vi "Ruler.vi"() -> ()   [LabVIEW 2023]
uses:
  <vilib>/measure/matone.llb/Extract Single Tone Information N Chan.vi
  <vilib>/express/express analysis/Spectral/Block/exnSpectralBlock spectral measurements RMS poly.vi
  <vilib>/express/express analysis/Spectral/Block/exnSpectralBlock spectral measurements RMS DDT.vi
  <vilib>/express/express analysis/Spectral/XNode/ExpressSpectralMeasurementsBlockNode.xnode
  <vilib>/measure/NI_MAPro.lvlib
panel:
  out "Waveform Chart of Acquired Sound":dynamicdata(graph) caption="Data"
  out "Fundamental Frequency as Sine Curve":dynamicdata(graph)
  out "FFT Waveform Graph":dynamicdata(graph)
  out "Detected Frequency (Hz)":dbl[](array[numeric]) format="%.2p"
  in  "Recording Duration (s)":dbl
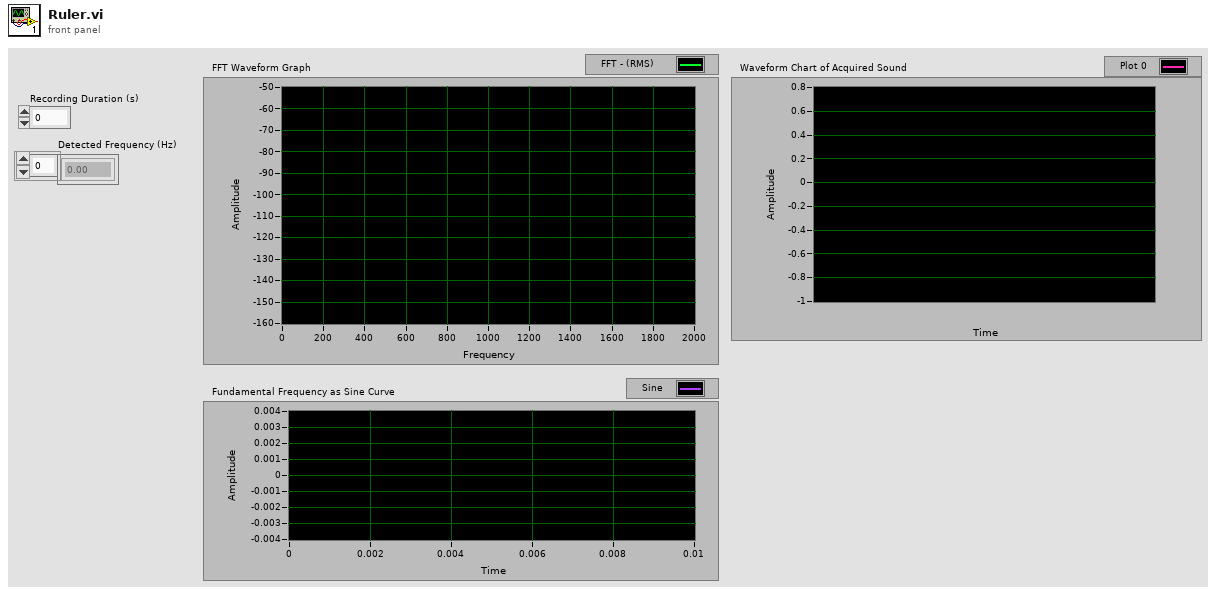
[diagram p1: front panel]
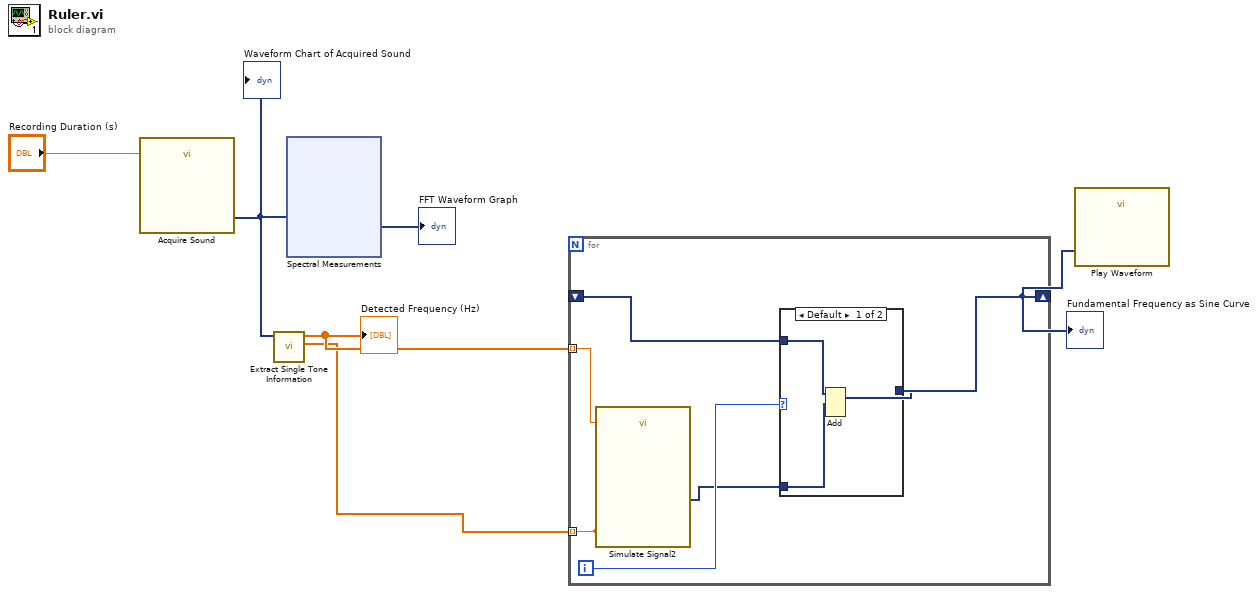
[diagram p0: block diagram]
diagram:
  n1 = call "Acquire Sound"("Duration (s)"="Recording Duration (s)") -> ("Data"=w2:dynamicdata)  [unwired: 17 in, 1 out]
  "Waveform Chart of Acquired Sound" <- w2
  n2 = call-poly <vilib>:"Extract Single Tone Information.vi"("time signals in"=w2) -> ("detected amplitudes"=w1:dbl[], "detected frequencies"=w3:dbl[])  [unwired: 5 in, 4 out]
  "Detected Frequency (Hz)" <- w3
  n3 = xnode "Spectral Measurements"("Signals"=w2) -> ("FFT - (RMS)"=→"FFT Waveform Graph":dynamicdata)  [unwired: 1 in, 2 out]
  n4 = for {
    tunnel: w3 -> [w12] mode=indexing
    shift-right: [w8] -> w4
    shift-left: _ -> [w11]
    tunnel: [w7] -> _ mode=indexing
    tunnel: w1 -> [w7] mode=indexing
    i -> [w10]
    n5 = call "Simulate Signal2"("Frequency"=w12, "Amplitude"=w7) -> ("Sine"=w9:dynamicdata)  [unwired: 12 in, 1 out]
    n6 = case shown="Default" w10 {
      tunnel: w9 -> [w15 w16]
      tunnel: w11 -> [w14 _]
      tunnel: [w13 w16] -> w8
      frame Default {
        n7 = Add(1:w15, 2:w14) -> (0:w13:dynamicdata)  [unwired: 1 in, 1 out]
      }
      frame 0 {
      }
    }
  }
  "Fundamental Frequency as Sine Curve" <- w4
  n8 = call "Play Waveform"("Data"=w4) -> ()  [unwired: 18 in, 1 out]
